vi "GetSpeed.vi"(8 "error in (no error)":errorcluster, 11 "Bike in":refnum<class "Bike.lvclass">) -> (0 "error out":errorcluster, 2 "speed":dbl, 3 "Bike out":refnum<class "Bike.lvclass">)   [LabVIEW 2019, in "Bike.lvclass"]
doc: "Gets the speed.\n\nwww.sciware.com.au"
uses:
  Bike.lvclass
  Bike.lvclass/Bike.ctl
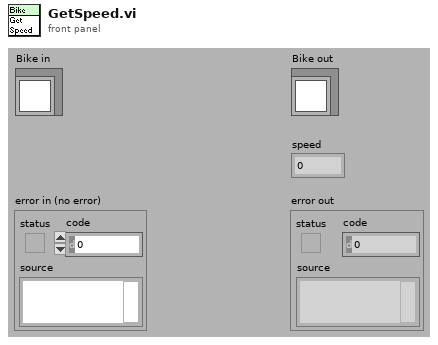
[diagram p1: front panel]
types:
  T1 = typedef "Bike.lvclass/DataRef.ctl" = refnum<data-value>
  T2 = typedef "Bike.lvclass/DataMembers.ctl" = cluster{"peddle rate":dbl}
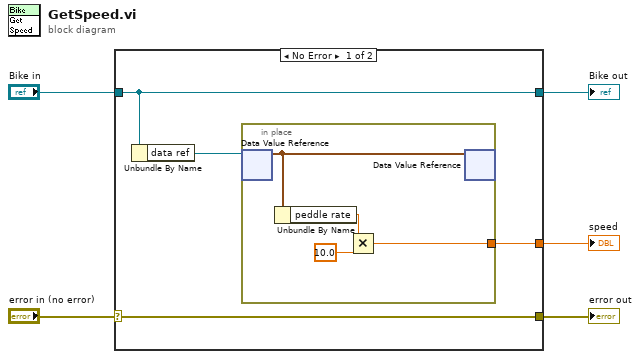
[diagram p0: block diagram]
diagram:
  n1 = case shown="No Error" "error in (no error)" {
    selector: "error in (no error)" -> [w9 w15]
    tunnel: [w9 w15] -> w4
    tunnel: [w8 w14] -> w2
    tunnel: "Bike in" -> [w8 w14]
    tunnel: [w6 _] -> w1
    frame No Error {
      n2 = Unbundle By Name(w8) -> ("data ref"=w7:T1)
      n3 = in-place {
        in-place-border: [w10] -> w6
        n4 = in-place-dvr #1(w7) -> (w13:T2)  [unwired: 1 out]
        n5 = Unbundle By Name(w13) -> ("peddle rate"=w12:dbl)
        n6 = Multiply(x=w12, y=10.0) -> (x*y=w10:dbl)
        n7 = in-place-dvr #1(w13) -> ()  [unwired: 2 out]
      }
    }
    frame Error {
    }
  }
  "error out" <- w4
  "Bike out" <- w2
  "speed" <- w1
